vi "logger.vi"(0 "new data":string, 1 "reset? (F)":bool) -> (6 "log data":string)   [LabVIEW 2018]
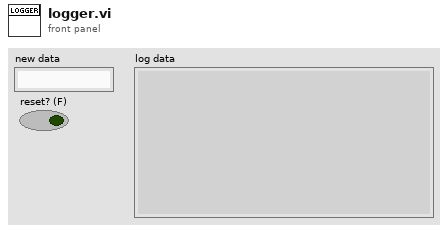
[diagram p1: front panel]
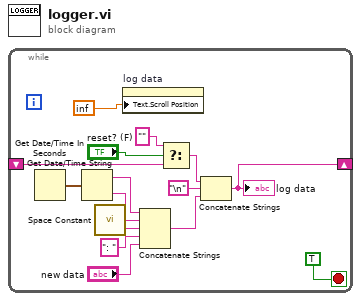
[diagram p0: block diagram]
diagram:
  n1 = while {
    shift-right: [w2] -> _
    shift-left: _ -> [w5]
    stop <- TRUE stop-if-true
    n2 = Get Date/Time In Seconds() -> (seconds since 1Jan1904=w11:timestamp)
    n3 = Get Date/Time String(seconds (now)=w11) -> (date string=w12:string, time string=w13:string)  [unwired: 2 in]
    n4 = call <vilib>:"Space Constant.vi"() -> ("String"=w14:string)
    n5 = property on="log data" class="Str"("Text.Scroll Position"=inf) -> ()  [unwired: 2 in, 2 out]
    n6 = Concatenate Strings(w12, w14, w13, ": " ("string"), "new data") -> (w8:string)
    n7 = Select(t="", s="reset? (F)", f=w5) -> (s? t:f=w4:string)
    n8 = Concatenate Strings(w4, "\n", w8) -> (w2:string)
    "log data" <- w2
  }
